vi "RepDoc Get Caption or Label Text.vi"(8 "error in (no error)":errorcluster, 11 "Ctl Refnum":refnum<vi>) -> (0 "error out":errorcluster, 2 "Caption or Label":string, 3 "Ctl Refnum out":refnum<vi>)   [LabVIEW 2020, in "NI_ReportGenerationCore.lvlib"]
doc: "Returns the Caption text for a control or indicator, if the caption exists. Otherwise returns the Label text."
uses:
  <vilib>/Utility/NIReport.llb/NI_ReportGenerationCore.lvlib
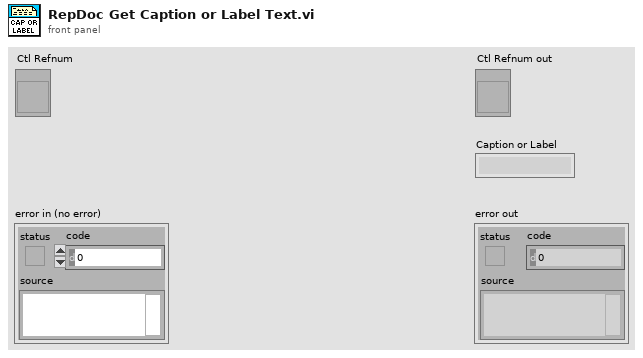
[diagram p1: front panel]
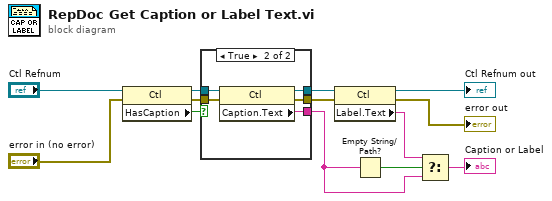
[diagram p0: block diagram]
diagram:
  n1 = property class="Ctl"(reference="Ctl Refnum", error in="error in (no error)") -> (reference out=w6:refnum<vi>, error out=w7:errorcluster, "HasCaption"=w13:bool)
  n2 = case shown="True" w13 {
    tunnel: w6 -> [w15 w20]
    tunnel: w7 -> [w14 w19]
    tunnel: [w15 w18] -> w9
    tunnel: [_ w17] -> w10
    tunnel: [w14 w16] -> w11
    frame False {
    }
    frame True {
      n3 = property class="Ctl"(reference=w20, error in=w19) -> (reference out=w18:refnum<vi>, error out=w16:errorcluster, "Caption.Text"=w17:string)
    }
  }
  n4 = property class="Ctl"(reference=w9, error in=w11) -> (reference out=→"Ctl Refnum out":refnum<vi>, error out=→"error out":errorcluster, "Label.Text"=w12:string)
  n5 = Empty String/Path?(string/path=w10) -> (empty?=w8:bool)
  n6 = Select(t=w12, s=w8, f=w10) -> (s? t:f=→"Caption or Label":string)
